vi "Fetch Binary I16.vi"(0 "device session in":refnum<class "Device Session.lvclass">, 1 "timeout (ms)":i32=10000, 5 "number of samples":u32=1000, 11 "error in":errorcluster) -> (4 "device session out":refnum<class "Device Session.lvclass">, 6 "target data out":i16[][](array[numeric]), 8 "scaling coefficients":cluster{"gain":dbl, "offset":dbl}[](array[cluster]), 10 "samples fetched":u32, 15 "error out":errorcluster)   [LabVIEW 2015, in "Device Session.lvclass"]
doc: "Fetches acquired samples and returns them in a two-dimensional array.\n\n<B>Input Parameters</B>\n\n<B>device session in</B> is a reference to the session containing sessions to all instrument design libraries used in this sample project. This parameter is obtained from the 'Open Session' VI.\n\n<B>number of samples</B> specifies the number of samples per channel to fetch. The default value is 1,000.\n\n<B>timeout (ms)</B> specifies the maximum amount of time to wait for the specified number of samples to be fetched. The default value is 10,000.\n\n<B>error in</B> describes error conditions that occur before this node runs. This input provides standard 'error in' functionality.\n\n<B>Output Parameters</B>\n\n<B>device session out</B> passes a reference to the session to the next VI.\n\n<B>target data out</B> returns a two-dimensional array with deinterleaved sample data.\n\n<B>scaling coefficients</B> returns an array of scaling coefficients for each streamed channel, which you can use to convert the returned data to Volts.\n\n<B>samples fetched</B> returns the number of samples per channel fetched.\n\n<B>error out</B> contains error information. This output provides standard 'error out' functionality."
uses:
  Device Session.lvclass
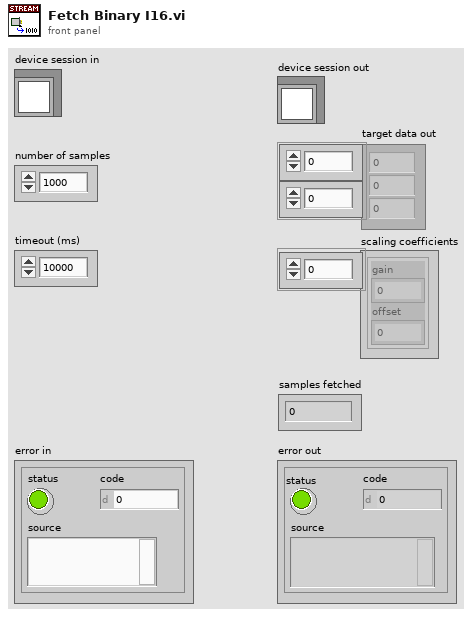
[diagram p1: front panel]
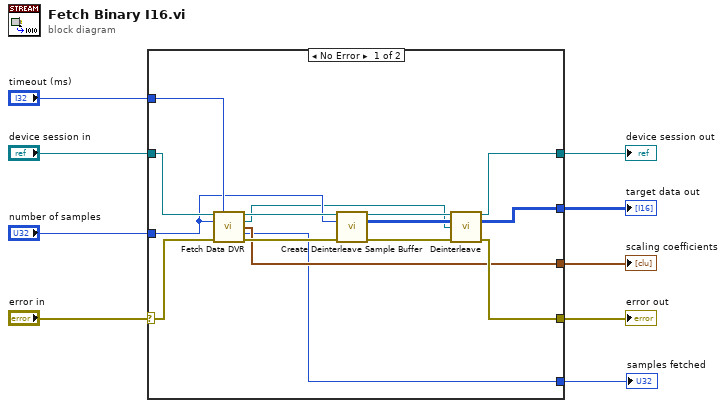
[diagram p0: block diagram]
diagram:
  n1 = case shown="No Error" "error in" {
    selector: "error in" -> [w18 w26]
    tunnel: [w15 w26] -> w8
    tunnel: [w21 w25] -> w7
    tunnel: "device session in" -> [w24 w25]
    tunnel: "timeout (ms)" -> [w20 _]
    tunnel: "number of samples" -> [w19 _]
    tunnel: [w14 _] -> w3
    tunnel: [w11 _] -> w2
    tunnel: [w10 _] -> w1
    frame No Error {
      n2 = call "Fetch Data DVR.vi"("device session in"=w24, "timeout (ms)"=w20, "number of samples"=w19, "error in"=w18) -> ("device session out"=w23:refnum<class "Device Session.lvclass">, "data"=w12:refnum<data-value>, "scaling coefficients"=w11:cluster{"gain":dbl, "offset":dbl}[], "samples fetched"=w10:u32, "error out"=w17:errorcluster)  [unwired: 7 in]
      n3 = call "Create Deinterleave Sample Buffer.vi"("device session in"=w23, "read size in samples"=w19, "error in"=w17) -> ("device session out"=w22:refnum<class "Device Session.lvclass">, "buffer"=w13:i16[][], "error out"=w16:errorcluster)  [unwired: 10 in]
      n4 = call "Deinterleave.vi"("device session in"=w22, "target data in"=w13, "source data"=w12, "error in"=w16) -> ("device session out"=w21:refnum<class "Device Session.lvclass">, "target data out"=w14:i16[][], "error out"=w15:errorcluster)  [unwired: 9 in]
    }
    frame Error {
    }
  }
  "target data out" <- w3
  "error out" <- w8
  "device session out" <- w7
  "scaling coefficients" <- w2
  "samples fetched" <- w1
